vi "Flock_ApplySysConfigException.vi"(8 "Error In":errorcluster, 11 "Process List":T1) -> (0 "Error Out":errorcluster)   [LabVIEW 2014, in "FA_ApplySysConfig.lvlib"]
uses:
  FA_ApplySysConfig.lvlib
  Shared Code/AMC/VI Source/CentralProcessMessaging/Flock_Shared_CentralProcessMessaging.lvlib
  Shared Code/AMC/VI Source/Error Handling/Flock_ErrorHandling.lvlib
  Shared Code/AMC/VI Source/LocalProcessMessaging/Flock_Shared_LocalProcessMessaging.lvlib
  Shared Code/AMC/VI Source/ProcessList.ctl
  Shared Code/AMC/VI Source/Flock_Shared_Messaging.lvlib
panel:
  out "resulting string":string
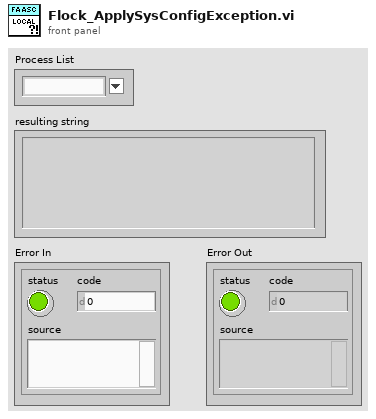
[diagram p1: front panel]
types:
  T1 = typedef "Flock_Shared_Messaging.lvlib/ProcessList.ctl" = string
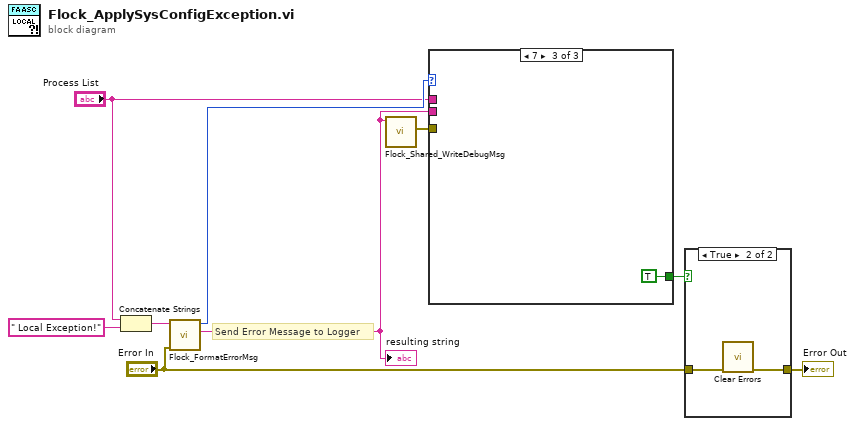
[diagram p0: block diagram]
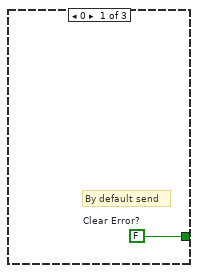
[diagram p3: hidden frame]
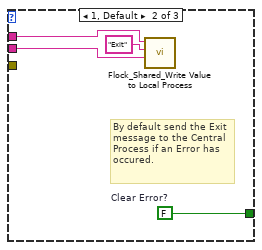
[diagram p4: hidden frame]
diagram:
  # "Send Error Message to Logger"
  n1 = Concatenate Strings("Process List", " Local Exception!" ("initial string")) -> (w1:string)
  n2 = call "Flock_FormatErrorMsg.vi"("error in (no error)"="Error In", "initial string"=w1) -> ("String"=w9:string, "code"=w8:i32)  [unwired: 8 in]
  "resulting string" <- w9
  n3 = call "Flock_Shared_WriteDebugMsg.vi"("Current Message Case"=w9) -> ("error out"=w4:errorcluster)  [unwired: 10 in]
  n4 = case shown="7" w8 {
    tunnel: w9 -> [_ w12 _]
    tunnel: [w10 w14 TRUE ("Clear Error?")] -> w7
    tunnel: w4 -> [_ _ _]
    tunnel: "Process List" -> [_ w13 _]
    frame 0 {
      w10 = FALSE  # Clear Error?
      # "By default send"
    }
    frame 1, Default {
      w14 = FALSE  # Clear Error?
      # "By default send the Exit message to the Central Process if an Error has occured."
      n5 = call "Flock_Shared_Write Value to Local Process.vi"("Message Value"=w12, "Message Name"="Exit", "Process List"=w13) -> ()  [unwired: 8 in, 1 out]
    }
    frame 7 {
    }
  }
  n6 = case shown="True" w7 {
    tunnel: "Error In" -> [w16 w18]
    tunnel: [w16 w17] -> w5
    frame False {
    }
    frame True {
      n7 = call <vilib>:"Clear Errors.vi"("error in (no error)"=w18) -> ("error out"=w17:errorcluster)  [unwired: 5 in, 1 out]
    }
  }
  "Error Out" <- w5
